vi "运维调试_五参数.vi"() -> ()   [LabVIEW 2016, in "斯坦道仪器.lvlib"]
uses:
  <vilib>/Utility/miscctls.llb/LVPointTypeDef.ctl
panel:
  out "COM口":string
  in  "打开串口":bool
  in  "释放串口":bool
  out "多参数横条运行状态":T1(xcontrol)
  in  "数据区":i32(listbox)
  in  "探头选择":u16(ring)=9 items=["氨氮"=3, "水温"=9, "pH值"=10, "溶解氧"=11, "电导率"=12, "浊度"=13, "叶绿素a"=14, "藻密度"=15, "蓝绿藻"=16, "氧化还原电位"=17, "溶解氧%"=18, "盐度"=19]
  in  "测量数据区读取":bool
  in  "测量数据区":i32(listbox)
  in  "状态告警区读取":bool
  in  "状态告警区":i32(listbox)
  in  "读取KB":bool
  in  "写入KB":bool
  out "B":dbl caption="校准值B:"
  out "K":dbl caption="校准值K:"
  in  "校准区探头选择":u16(ring)=9 items=["氨氮"=3, "水温"=9, "pH值"=10, "溶解氧"=11, "电导率"=12, "浊度"=13, "叶绿素a"=14, "藻密度"=15, "蓝绿藻"=16, "氧化还原电位"=17, "溶解氧%"=18, "盐度"=19]
  in  "停止测量(单探)":bool
  in  "启动测量(单探)":bool
  in  "控制命令区探头选择":u16(ring)=9 items=["氨氮"=3, "水温"=9, "pH值"=10, "溶解氧"=11, "电导率"=12, "浊度"=13, "叶绿素a"=14, "藻密度"=15, "蓝绿藻"=16, "氧化还原电位"=17, "溶解氧%"=18, "盐度"=19]
  in  "同步时间":bool
  in  "初始化(清洗)":bool
  in  "停止测量(全部)":bool
  in  "启动测量(全部)":bool
  in  "关键参数区读取":bool
  in  "关键参数区":i32(listbox)
  in  "传感器参数读取":bool
  in  "传感器区":i32(listbox)
  in  "返回":bool
  in  "设置":bool
  out "运行状态":string
  out "开机状态":bool
  in  "停止":bool
  in  "手动启动":bool
  out "集成报警信息":string
  # "控制命令区"
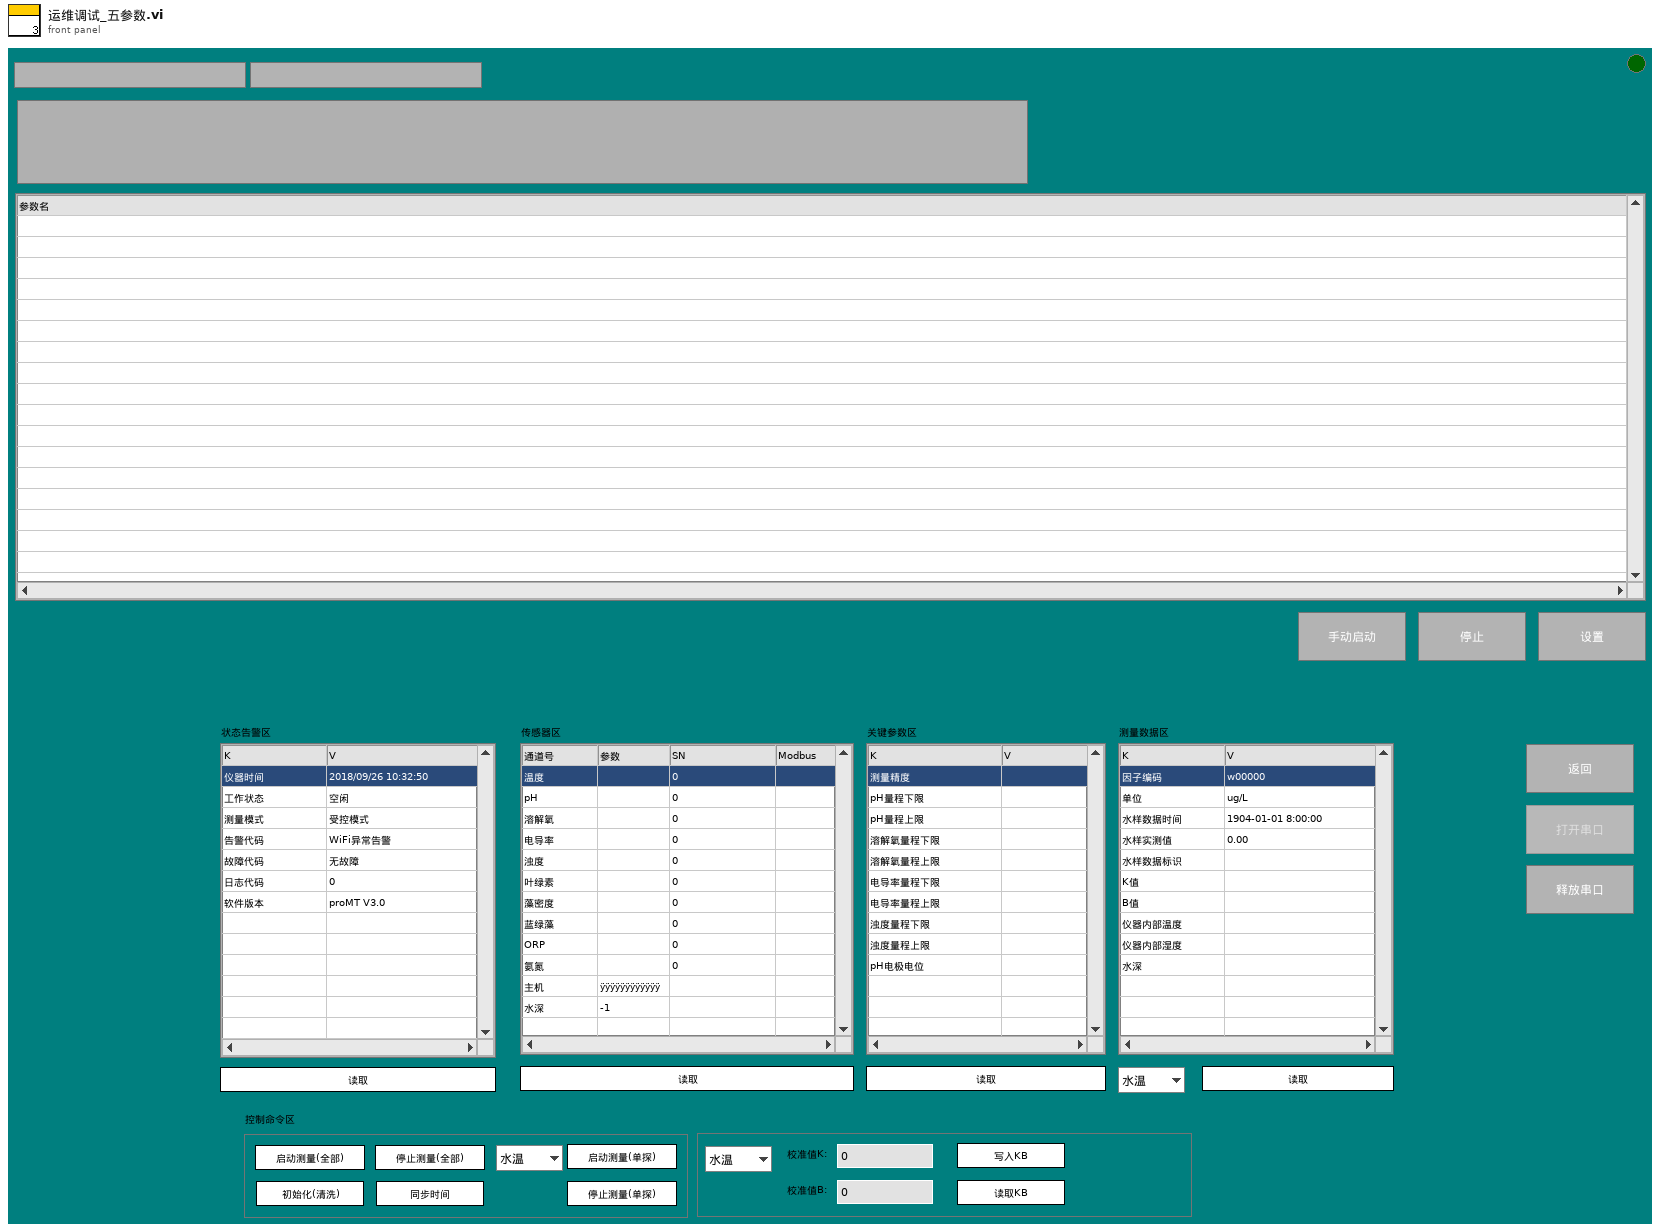
[diagram p1: front panel]
types:
  T1 = cluster{"系统时间":timestamp, "工作状态":u16, "测量模式":u16, "告警代码":enum16{"无告警", "缺试剂告警", "缺水样告警", "缺蒸馏水告警", "缺标液告警", "仪表漏液告警", "标定异常告警", "超量程告警", "加热异常", "低试剂预警", "超上限告警", "超下限告警", "仪表内部其他异常", "滴定异常告警", "电极异常告警", "量程切换告警", "参数设置告警", "PH电极电位异常", "电导率电极异常", "浊度光度异常", "溶解氧电极异常", "溶解氧光强异常", "温度异常告警", "PH异常告警", "溶解氧异常告警", "电导率异常告警", "浊度异常告警", "叶绿素异常告警", "藻密度异常告警", "蓝绿藻异常告警", "ORP异常告警", "氨氮异常告警", "清洁刷异常告警", "SD卡异常告警", "蓝牙异常告警", "Wifi异常告警", "流程异常告警"}, "故障代码":enum16{"无故障", "电机故障", "温度故障", "通讯故障", "滴定故障"}, "日志代码":u16, "软件版本":string}
  T2 = typedef "LVPointTypeDef.ctl" = cluster{"Horizontal":i16, "Vertical":i16}
  T3 = cluster{"时间标识":timestamp, "设备":string, "日志信息":string}
  T4 = enum16{"无告警", "缺试剂告警", "缺水样告警", "缺蒸馏水告警", "缺标液告警", "仪表漏液告警", "标定异常告警", "超量程告警", "加热异常", "低试剂预警", "超上限告警", "超下限告警", "仪表内部其他异常", "滴定异常告警", "电极异常告警", "量程切换告警", "参数设置告警", "PH电极电位异常", "电导率电极异常", "浊度光度异常", "溶解氧电极异常", "溶解氧光强异常", "温度异常告警", "PH异常告警", "溶解氧异常告警", "电导率异常告警", "浊度异常告警", "叶绿素异常告警", "藻密度异常告警", "蓝绿藻异常告警", "ORP异常告警", "氨氮异常告警", "清洁刷异常告警", "SD卡异常告警", "蓝牙异常告警", "Wifi异常告警", "流程异常告警"}
  T5 = cluster{"水温":dbl, "pH":dbl, "DO":dbl, "Cond":dbl, "Turb":dbl, "叶绿素":dbl, "藻密度":dbl, "蓝绿藻":dbl, "ORP":dbl, "NH3N":dbl}
  T6 = cluster{"因子编码":string, "单位":string, "标样参考值":sgl, "水样数据时间":timestamp, "水样实测值":sgl, "水样数据标识":string, "K":sgl, "B":sgl, "T":sgl, "H":sgl, "水深":sgl, "探头温度":sgl}
  T7 = enum8{"Enabled", "Disabled", "Disabled and Grayed Out"}
  T8 = cluster{"测量模式":enum16{"待机", "水样测试", "标样核查", "零点核查", "跨度核查", "空白测试", "平行样测试", "加标回收", "空白校准", "标样校准", "初始化（清洗）"}, "数据标记表":string, "测量时间":dbl}
  T9 = enum32{"Bad", "Idle", "Run top level", "Running"}
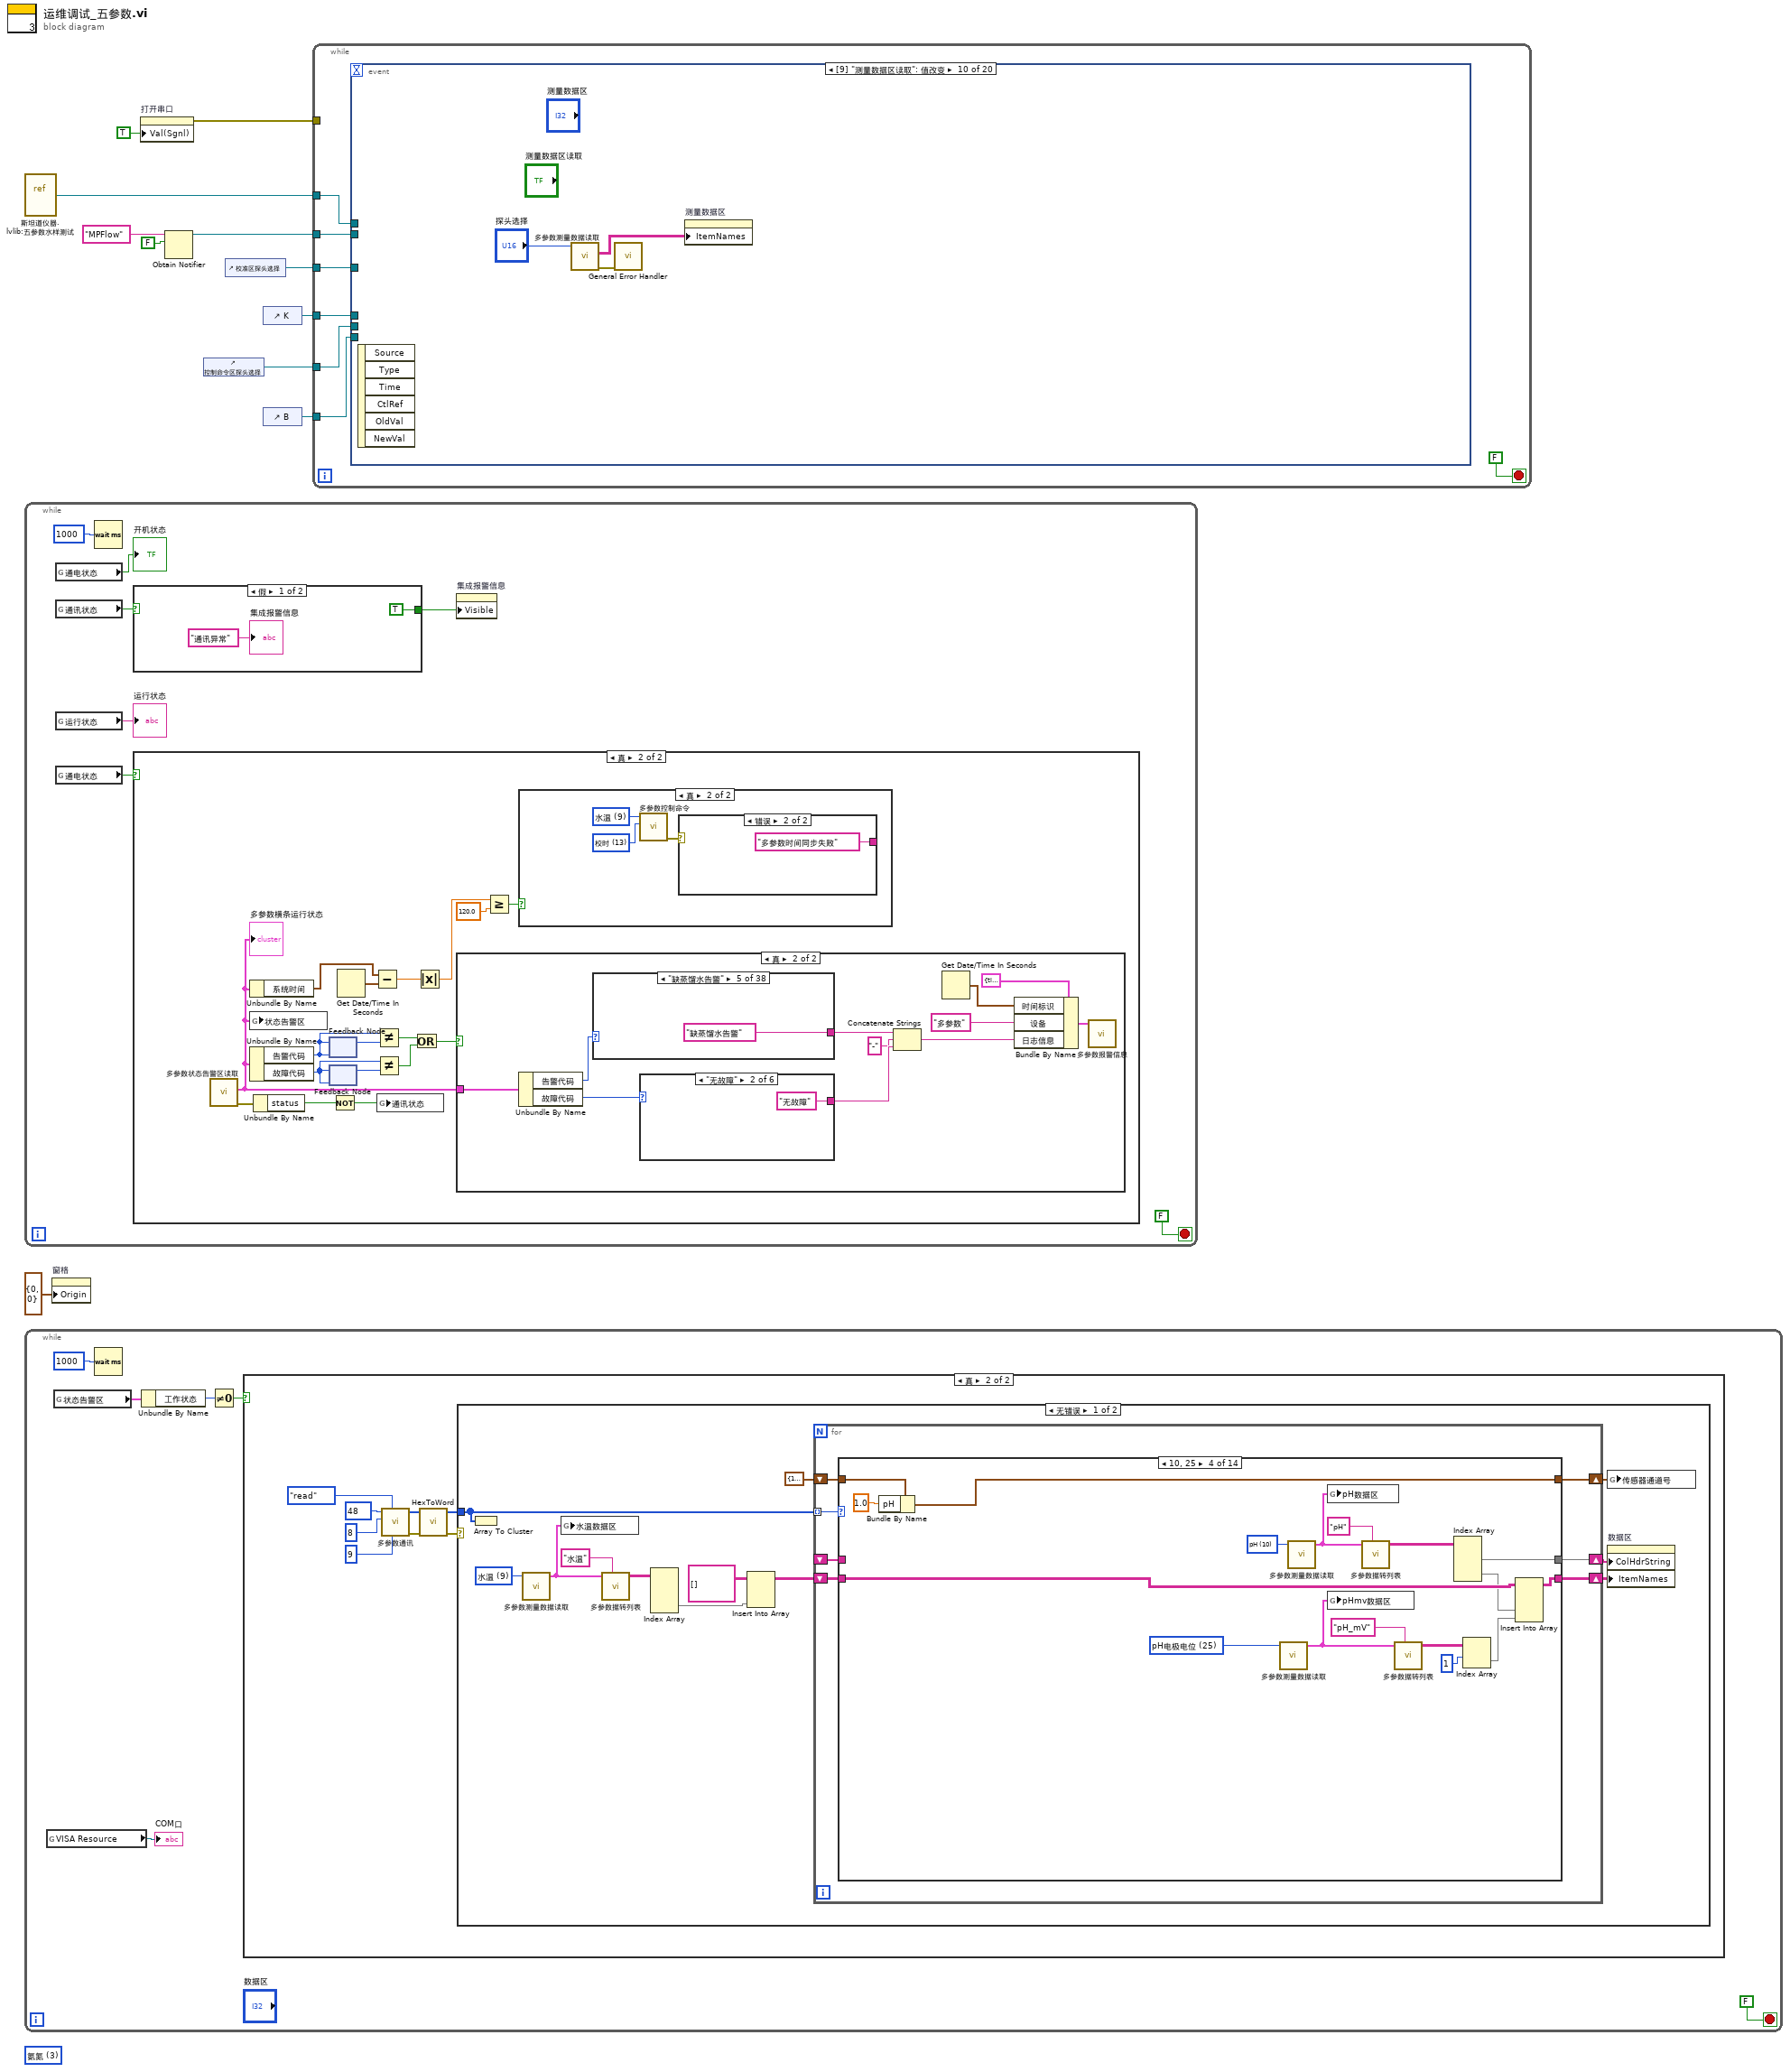
[diagram p0: block diagram]
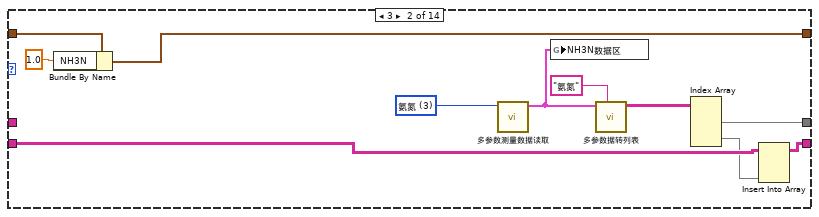
[diagram p4: hidden frame]
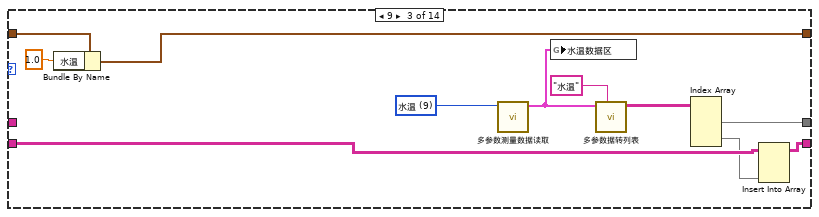
[diagram p5: hidden frame]
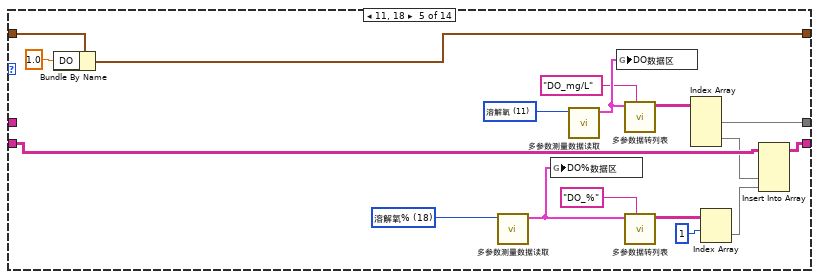
[diagram p6: hidden frame]
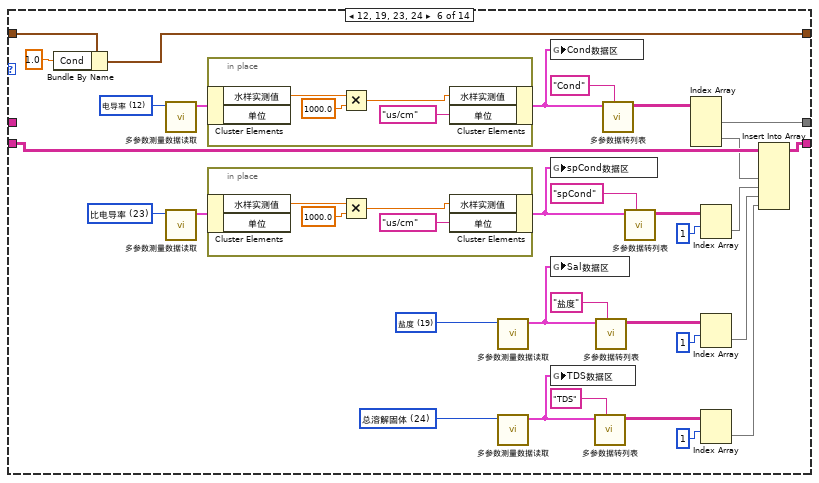
[diagram p7: hidden frame]
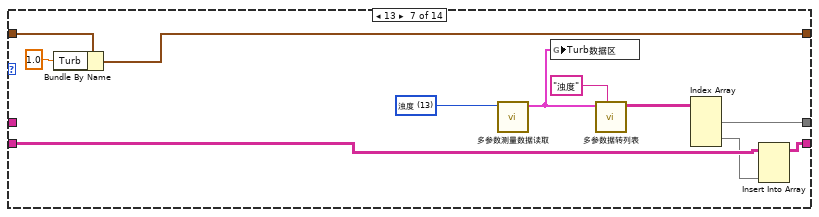
[diagram p8: hidden frame]
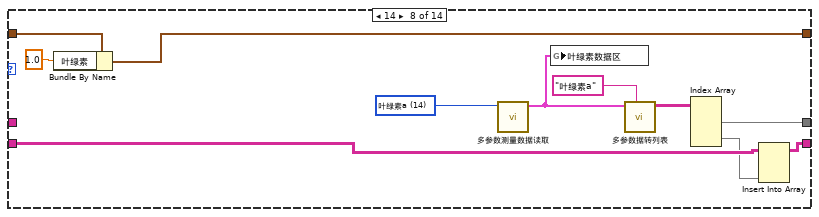
[diagram p9: hidden frame]
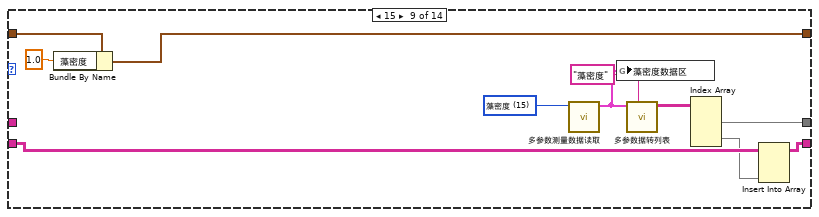
[diagram p10: hidden frame]
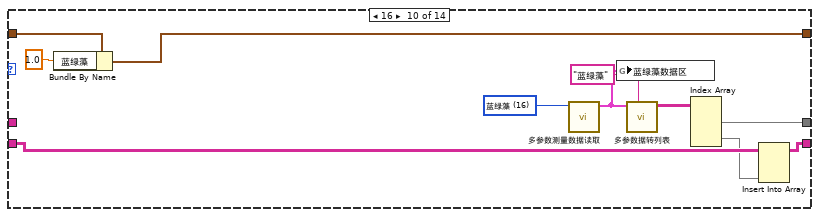
[diagram p11: hidden frame]
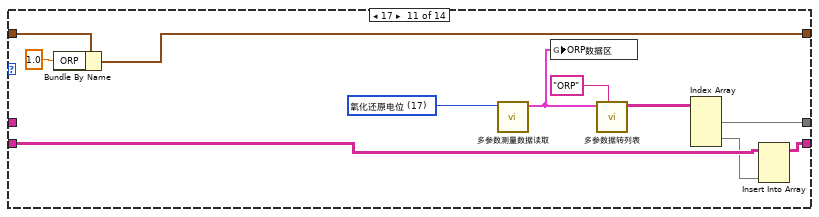
[diagram p12: hidden frame]
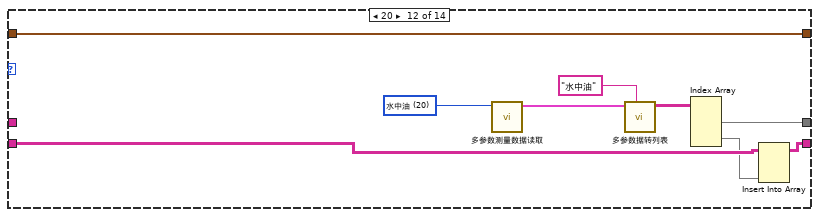
[diagram p13: hidden frame]
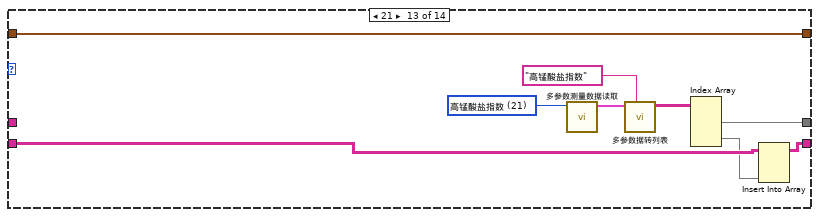
[diagram p14: hidden frame]
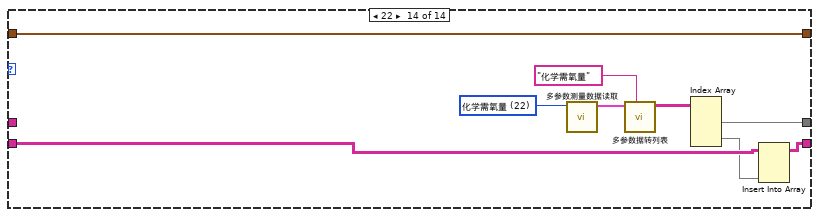
[diagram p15: hidden frame]
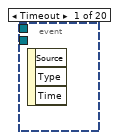
[diagram p17: hidden frame]
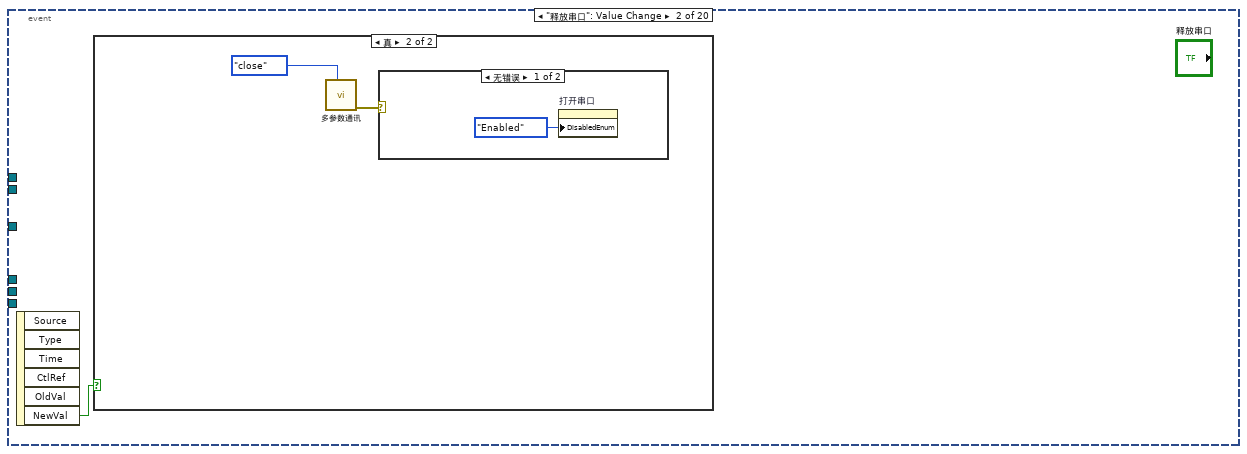
[diagram p18: hidden frame]
diagram:
  (unwired) u16 3 items=["氨氮"=3, "水温"=9, "pH"=10, "溶解氧"=11, "电导率"=12, "浊度"=13, "叶绿素a"=14, "藻密度"=15, "蓝绿藻"=16, "氧化还原电位"=17, "溶解氧%"=18, "盐度"=19, "水中油"=20, "高锰酸盐指数"=21, "化学需氧量"=22, "比电导率"=23, "总溶解固体"=24, "pH电极电位"=25] ("下拉列表")
  n1 = vi-ref "斯坦道仪器.lvlib:五参数水样测试.vi"() -> (w8:refnum<vi>)
  n2 = while {
    stop <- FALSE stop-if-true
    n3 = global read "多参数全局变量.vi" "通电状态"() -> (→"开机状态":bool)
    n4 = global read "多参数全局变量.vi" "通讯状态"() -> (w16:bool)
    n5 = global read "多参数全局变量.vi" "运行状态"() -> (→"运行状态":string)
    n6 = global read "多参数全局变量.vi" "通电状态"() -> (w12:bool)
    n7 = Wait (ms)(milliseconds to wait=u32 1000 ("等待时间（毫秒）")) -> ()  [unwired: 1 out]
    n8 = case shown="假" w16 {
      tunnel: [TRUE ("可见") _] -> w15
      frame False {
        "集成报警信息" <- "通讯异常" ("集成报警信息")
      }
      frame True {
      }
    }
    n9 = case shown="真" w12 {
      frame False {
      }
      frame True {
        n10 = call "多参数状态告警区读取.vi"() -> ("error out"=w28:errorcluster, "状态告警块"=w25:T1)  [unwired: 9 in, 1 out]
        "多参数横条运行状态" <- w25
        n11 = Unbundle By Name(w25) -> ("系统时间"=w24:timestamp)
        n12 = global write "多参数全局变量.vi" "状态告警区"(w25) -> ()
        n13 = Unbundle By Name(w25) -> ("告警代码"=w34:T4, "故障代码"=w32:enum16{"无故障", "电机故障", "温度故障", "通讯故障", "滴定故障"})
        n14 = Unbundle By Name(w28) -> ("status"=w27:bool)
        n15 = feedback #1(w34) -> (w35:T4)
        n16 = feedback-in #1(w34) -> ()
        n17 = feedback #2(w32) -> (w33:enum16{"无故障", "电机故障", "温度故障", "通讯故障", "滴定故障"})
        n18 = feedback-in #2(w32) -> ()
        n19 = Not(x=w27) -> (.not. x?=w26:bool)
        n20 = Get Date/Time In Seconds() -> (seconds since 1Jan1904=w23:timestamp)
        n21 = Subtract(x=w24, y=w23) -> (x-y=w22:dbl)
        n22 = Not Equal?(x=w34, y=w35) -> (x != y?=w30:bool)
        n23 = Not Equal?(x=w32, y=w33) -> (x != y?=w31:bool)
        n24 = global write "多参数全局变量.vi" "通讯状态"(w26) -> ()
        n25 = Or(x=w30, y=w31) -> (x .or. y?=w29:bool)
        n26 = Absolute Value(x=w22) -> (abs(x)=w21:dbl)
        n27 = case shown="真" w29 {
          tunnel: w25 -> [_ w51]
          frame False {
          }
          frame True {
            n28 = Unbundle By Name(w51) -> ("告警代码"=w50:T4, "故障代码"=w49:enum16{"无故障", "电机故障", "温度故障", "通讯故障", "滴定故障"})
            n29 = case shown="\"缺蒸馏水告警\"" w50 {
              selector: w50 -> [w62 _ _ _ _ _ _ _ _ _ _ _ _ _ _ _ _ _ _ _ _ _ _ _ _ _ _ _ _ _ _ _ _ _ _ _ _ _]
              tunnel: [w61 "无告警" "缺试剂告警" "缺水样告警" "缺蒸馏水告警" "缺标液告警" "仪表漏液告警" "标定异常告警" "超量程告警" "加热异常" "低试剂预警" "超上限告警" "超下限告警" "仪表内部其他异常" "滴定异常告警" "电极异常告警" "量程切换告警" "参数设置告警" "PH电极电位异常" "电导率电极异常" "浊度光度异常" "溶解氧电极异常" "溶解氧光强异常" "温度异常告警" "PH异常告警" "溶解氧异常告警" "电导率异常告警" "浊度异常告警" "叶绿素异常告警" "藻密度异常告警" "蓝绿藻异常告警" "ORP异常告警" "氨氮异常告警" "清洁刷异常告警" "SD卡异常告警" "蓝牙异常告警" "WiFi异常告警" "流程异常告警"] -> w48
              frame Default {
                n30 = Format Into String(format string="%d" ("格式字符串"), initial string="未知" ("工作状态"), w62) -> (resulting string=w61:string)  [unwired: 1 in, 1 out]
              }
              frame "无告警" {
              }
              frame "缺试剂告警" {
              }
              frame "缺水样告警" {
              }
              frame "缺蒸馏水告警" {
              }
              frame "缺标液告警" {
              }
              frame "仪表漏液告警" {
              }
              frame "标定异常告警" {
              }
              frame "超量程告警" {
              }
              frame "加热异常" {
              }
              frame "低试剂预警" {
              }
              frame "超上限告警" {
              }
              frame "超下限告警" {
              }
              frame "仪表内部其他异常" {
              }
              frame "滴定异常告警" {
              }
              frame "电极异常告警" {
              }
              frame "量程切换告警" {
              }
              frame "参数设置告警" {
              }
              frame "PH电极电位异常" {
              }
              frame "电导率电极异常" {
              }
              frame "浊度光度异常" {
              }
              frame "溶解氧电极异常" {
              }
              frame "溶解氧光强异常" {
              }
              frame "温度异常告警" {
              }
              frame "PH异常告警" {
              }
              frame "溶解氧异常告警" {
              }
              frame "电导率异常告警" {
              }
              frame "浊度异常告警" {
              }
              frame "叶绿素异常告警" {
              }
              frame "藻密度异常告警" {
              }
              frame "蓝绿藻异常告警" {
              }
              frame "ORP异常告警" {
              }
              frame "氨氮异常告警" {
              }
              frame "清洁刷异常告警" {
              }
              frame "SD卡异常告警" {
              }
              frame "蓝牙异常告警" {
              }
              frame "Wifi异常告警" {
              }
              frame "流程异常告警" {
              }
            }
            n31 = case shown="\"无故障\"" w49 {
              selector: w49 -> [w53 _ _ _ _ _]
              tunnel: [w52 "无故障" "电机故障" "温度故障" "通讯故障" "滴定故障"] -> w47
              frame Default {
                n32 = Format Into String(format string="%d" ("格式字符串"), initial string="未知" ("工作状态"), w53) -> (resulting string=w52:string)  [unwired: 1 in, 1 out]
              }
              frame "无故障" {
              }
              frame "电机故障" {
              }
              frame "温度故障" {
              }
              frame "通讯故障" {
              }
              frame "滴定故障" {
              }
            }
            n33 = Concatenate Strings(w48, "-" ("字符串"), w47) -> (w43:string)
            n34 = Get Date/Time In Seconds() -> (seconds since 1Jan1904=w42:timestamp)
            n35 = Bundle By Name(cluster=T3 {"时间标识"=timestamp(0 s since 1904-01-01), "设备"="", "日志信息"=""} ("data in"), "时间标识"=w42, "设备"="多参数", "日志信息"=w43) -> (w44:T3)
            n36 = call "多参数报警信息.vi"("data in"=w44) -> ()  [unwired: 10 in, 1 out]
          }
        }
        n37 = Greater Or Equal?(x=w21, y=120.0) -> (x >= y?=w20:bool)
        n38 = case shown="真" w20 {
          frame False {
          }
          frame True {
            w36 = u16 13 items=["启动测量（全部）"=1, "初始化（清洗）"=10, "停止测量（全部）"=11, "校时"=13, "启动测量（单个传感器）"=19, "停止测量（单个传感器）"=20] ("控制命令")
            w37 = u16 9 items=["氨氮"=3, "水温"=9, "pH值"=10, "溶解氧"=11, "电导率"=12, "浊度"=13, "叶绿素a"=14, "藻密度"=15, "蓝绿藻"=16, "氧化还原电位"=17, "溶解氧%"=18, "盐度"=19] ("站号")
            n39 = call "多参数控制命令.vi"("控制命令"=w36, "站号"=w37) -> ("error out"=w38:errorcluster)  [unwired: 9 in]
            n40 = case shown="错误" w38 {
              tunnel: ["多参数时间同步成功" ("消息") "多参数时间同步失败" ("消息")] -> _
              frame No Error {
              }
              frame Error {
              }
            }
          }
        }
      }
    }
    n41 = property on="集成报警信息" class="Str"("Visible"=w15) -> ()  [unwired: 2 in, 2 out]
  }
  n42 = while {
    stop <- FALSE stop-if-true
    n43 = global read "多参数全局变量.vi" "VISA Resource"() -> (→"COM口":refnum<visa-resource-name>)
    n44 = global read "多参数全局变量.vi" "状态告警区"() -> (w107:T1)
    n45 = Wait (ms)(milliseconds to wait=u32 1000 ("等待时间（毫秒）")) -> ()  [unwired: 1 out]
    n46 = Unbundle By Name(w107) -> ("工作状态"=w106:u16)
    n47 = Not Equal To 0?(x=w106) -> (x != 0?=w105:bool)
    n48 = case shown="真" w105 {
      frame False {
      }
      frame True {
        n49 = call "多参数通讯.vi"("Slave ID"=u8 9, "STEP"=enum16{"open", "read", "write", "close"}."read", "quantity"=u16 8, "starting address"=u16 48) -> ("error out"=w112:errorcluster, "Registers"=w113:u16[])  [unwired: 5 in, 1 out]
        n50 = call "HexToWord.vi"("数组"=w113) -> ("WORD"=w116:u16[])  [unwired: 10 in]
        n51 = case shown="无错误" w112 {
          tunnel: w116 -> [w128 _]
          frame No Error {
            w125 = u16 9 items=["氨氮"=3, "水温"=9, "pH"=10, "溶解氧"=11, "电导率"=12, "浊度"=13, "叶绿素a"=14, "藻密度"=15, "蓝绿藻"=16, "氧化还原电位"=17, "溶解氧%"=18, "盐度"=19, "水中油"=20, "高锰酸盐指数"=21, "化学需氧量"=22, "比电导率"=23, "总溶解固体"=24, "pH电极电位"=25] ("下拉列表")
            n52 = Array To Cluster(array=w128) -> ()  [unwired: 1 out]
            n53 = call "多参数测量数据读取.vi"("探头选择"=w125) -> ("测量数据块"=w120:T6)  [unwired: 8 in, 2 out]
            n54 = global write "多参数全局变量.vi" "水温数据区"(w120) -> ()
            n55 = call "多参数据转列表.vi"("参数名"="水温", "测量数据块"=w120) -> ("添加的数组"=w118:string[][])  [unwired: 9 in]
            n56 = Index Array(array=w118) -> (element #2=w117:string[])  [unwired: 4 in, 1 out]
            n57 = Insert Into Array(array=string[][] [] ("子数组"), new element=w117) -> (w123:string[][])  [unwired: 2 in]
            n58 = for {
              tunnel: w128 -> [w135] mode=indexing
              shift-right: [w133] -> w126
              shift-left: w123 -> [w134]
              shift-right: [w132] -> w127
              shift-left: _ -> [w131]
              shift-right: [w130] -> w121
              shift-left: T5 {"水温"=1.0, "pH"=0.0, "DO"=0.0, "Cond"=0.0, "Turb"=0.0, "叶绿素"=0.0, "藻密度"=0.0, "蓝绿藻"=0.0, "ORP"=0.0, "NH3N"=0.0} ("传感器通道号") -> [w129]
              n59 = case shown="10, 25" w135 {
                tunnel: w134 -> [w138 w148 w159 w176 w193 w224 w243 w254 w265 w276 w287 w296 w305 w314]
                tunnel: [w138 w147 w158 w175 w192 w223 w242 w253 w264 w275 w286 w295 w304 w313] -> w133
                tunnel: [w137 w140 w151 w168 w185 w214 w236 w246 w259 w269 w280 w290 w299 w308] -> w132
                tunnel: w131 -> [w137 _ _ _ _ _ _ _ _ _ _ _ _ _]
                tunnel: [w136 w144 w155 w171 w189 w217 w239 w250 w261 w272 w283 w294 w303 w312] -> w130
                tunnel: w129 -> [w136 w146 w157 w173 w191 w218 w240 w251 w262 w273 w284 w294 w303 w312]
                frame 0, Default {
                }
                frame 3 {
                  w149 = u16 3 items=["氨氮"=3, "水温"=9, "pH"=10, "溶解氧"=11, "电导率"=12, "浊度"=13, "叶绿素a"=14, "藻密度"=15, "蓝绿藻"=16, "氧化还原电位"=17, "溶解氧%"=18, "盐度"=19, "水中油"=20, "高锰酸盐指数"=21, "化学需氧量"=22, "比电导率"=23, "总溶解固体"=24, "pH电极电位"=25] ("下拉列表")
                  n60 = Bundle By Name(cluster=w146, "NH3N"=1.0) -> (w144:T5)
                  n61 = call "多参数测量数据读取.vi"("探头选择"=w149) -> ("测量数据块"=w143:T6)  [unwired: 8 in, 2 out]
                  n62 = global write "多参数全局变量.vi" "NH3N数据区"(w143) -> ()
                  n63 = call "多参数据转列表.vi"("参数名"="氨氮", "测量数据块"=w143) -> ("添加的数组"=w142:string[][])  [unwired: 9 in]
                  n64 = Index Array(array=w142) -> (element #1=w140:string[], element #2=w139:string[])  [unwired: 4 in]
                  n65 = Insert Into Array(array=w148, new element=w139) -> (w147:string[][])  [unwired: 2 in]
                }
                frame 9 {
                  w160 = u16 9 items=["氨氮"=3, "水温"=9, "pH"=10, "溶解氧"=11, "电导率"=12, "浊度"=13, "叶绿素a"=14, "藻密度"=15, "蓝绿藻"=16, "氧化还原电位"=17, "溶解氧%"=18, "盐度"=19, "水中油"=20, "高锰酸盐指数"=21, "化学需氧量"=22, "比电导率"=23, "总溶解固体"=24, "pH电极电位"=25] ("下拉列表")
                  n66 = Bundle By Name(cluster=w157, "水温"=1.0) -> (w155:T5)
                  n67 = call "多参数测量数据读取.vi"("探头选择"=w160) -> ("测量数据块"=w154:T6)  [unwired: 8 in, 2 out]
                  n68 = global write "多参数全局变量.vi" "水温数据区"(w154) -> ()
                  n69 = call "多参数据转列表.vi"("参数名"="水温", "测量数据块"=w154) -> ("添加的数组"=w153:string[][])  [unwired: 9 in]
                  n70 = Index Array(array=w153) -> (element #1=w151:string[], element #2=w150:string[])  [unwired: 4 in]
                  n71 = Insert Into Array(array=w159, new element=w150) -> (w158:string[][])  [unwired: 2 in]
                }
                frame 10, 25 {
                  w174 = u16 25 items=["氨氮"=3, "水温"=9, "pH"=10, "溶解氧"=11, "电导率"=12, "浊度"=13, "叶绿素a"=14, "藻密度"=15, "蓝绿藻"=16, "氧化还原电位"=17, "溶解氧%"=18, "盐度"=19, "水中油"=20, "高锰酸盐指数"=21, "化学需氧量"=22, "比电导率"=23, "总溶解固体"=24, "pH电极电位"=25] ("下拉列表")
                  w177 = u16 10 items=["氨氮"=3, "水温"=9, "pH"=10, "溶解氧"=11, "电导率"=12, "浊度"=13, "叶绿素a"=14, "藻密度"=15, "蓝绿藻"=16, "氧化还原电位"=17, "溶解氧%"=18, "盐度"=19, "水中油"=20, "高锰酸盐指数"=21, "化学需氧量"=22, "比电导率"=23, "总溶解固体"=24, "pH电极电位"=25] ("下拉列表")
                  n72 = Bundle By Name(cluster=w173, "pH"=1.0) -> (w171:T5)
                  n73 = call "多参数测量数据读取.vi"("探头选择"=w174) -> ("测量数据块"=w164:T6)  [unwired: 8 in, 2 out]
                  n74 = call "多参数测量数据读取.vi"("探头选择"=w177) -> ("测量数据块"=w170:T6)  [unwired: 8 in, 2 out]
                  n75 = global write "多参数全局变量.vi" "pH数据区"(w170) -> ()
                  n76 = global write "多参数全局变量.vi" "pHmv数据区"(w164) -> ()
                  n77 = call "多参数据转列表.vi"("参数名"="pH", "测量数据块"=w170) -> ("添加的数组"=w169:string[][])  [unwired: 9 in]
                  n78 = call "多参数据转列表.vi"("参数名"="pH_mV", "测量数据块"=w164) -> ("添加的数组"=w163:string[][])  [unwired: 9 in]
                  n79 = Index Array(array=w169) -> (element #1=w168:string[], element #2=w167:string[])  [unwired: 4 in]
                  n80 = Index Array(array=w163, index (row)=1 ("禁用的索引 (列)")) -> (element=w166:string[])  [unwired: 1 in]
                  n81 = Insert Into Array(array=w176, new element #1=w167, new element #2=w166) -> (w175:string[][])  [unwired: 2 in]
                }
                frame 11, 18 {
                  w183 = u16 18 items=["氨氮"=3, "水温"=9, "pH"=10, "溶解氧"=11, "电导率"=12, "浊度"=13, "叶绿素a"=14, "藻密度"=15, "蓝绿藻"=16, "氧化还原电位"=17, "溶解氧%"=18, "盐度"=19, "水中油"=20, "高锰酸盐指数"=21, "化学需氧量"=22, "比电导率"=23, "总溶解固体"=24, "pH电极电位"=25] ("下拉列表")
                  w194 = u16 11 items=["氨氮"=3, "水温"=9, "pH"=10, "溶解氧"=11, "电导率"=12, "浊度"=13, "叶绿素a"=14, "藻密度"=15, "蓝绿藻"=16, "氧化还原电位"=17, "溶解氧%"=18, "盐度"=19, "水中油"=20, "高锰酸盐指数"=21, "化学需氧量"=22, "比电导率"=23, "总溶解固体"=24, "pH电极电位"=25] ("下拉列表")
                  n82 = Bundle By Name(cluster=w191, "DO"=1.0) -> (w189:T5)
                  n83 = call "多参数测量数据读取.vi"("探头选择"=w183) -> ("测量数据块"=w182:T6)  [unwired: 8 in, 2 out]
                  n84 = global write "多参数全局变量.vi" "DO%数据区"(w182) -> ()
                  n85 = call "多参数测量数据读取.vi"("探头选择"=w194) -> ("测量数据块"=w188:T6)  [unwired: 8 in, 2 out]
                  n86 = global write "多参数全局变量.vi" "DO数据区"(w188) -> ()
                  n87 = call "多参数据转列表.vi"("参数名"="DO_mg/L", "测量数据块"=w188) -> ("添加的数组"=w186:string[][])  [unwired: 9 in]
                  n88 = call "多参数据转列表.vi"("参数名"="DO_%", "测量数据块"=w182) -> ("添加的数组"=w180:string[][])  [unwired: 9 in]
                  n89 = Index Array(array=w186) -> (element #1=w185:string[], element #2=w184:string[])  [unwired: 4 in]
                  n90 = Index Array(array=w180, index (row)=1 ("禁用的索引 (列)")) -> (element=w179:string[])  [unwired: 1 in]
                  n91 = Insert Into Array(array=w193, new element #1=w184, new element #2=w179) -> (w192:string[][])  [unwired: 2 in]
                }
                frame 12, 19, 23, 24 {
                  w220 = u16 24 items=["氨氮"=3, "水温"=9, "pH"=10, "溶解氧"=11, "电导率"=12, "浊度"=13, "叶绿素a"=14, "藻密度"=15, "蓝绿藻"=16, "氧化还原电位"=17, "溶解氧%"=18, "盐度"=19, "水中油"=20, "高锰酸盐指数"=21, "化学需氧量"=22, "比电导率"=23, "总溶解固体"=24, "pH电极电位"=25] ("下拉列表")
                  w221 = u16 19 items=["氨氮"=3, "水温"=9, "pH"=10, "溶解氧"=11, "电导率"=12, "浊度"=13, "叶绿素a"=14, "藻密度"=15, "蓝绿藻"=16, "氧化还原电位"=17, "溶解氧%"=18, "盐度"=19, "水中油"=20, "高锰酸盐指数"=21, "化学需氧量"=22, "比电导率"=23, "总溶解固体"=24, "pH电极电位"=25] ("下拉列表")
                  w222 = u16 23 items=["氨氮"=3, "水温"=9, "pH"=10, "溶解氧"=11, "电导率"=12, "浊度"=13, "叶绿素a"=14, "藻密度"=15, "蓝绿藻"=16, "氧化还原电位"=17, "溶解氧%"=18, "盐度"=19, "水中油"=20, "高锰酸盐指数"=21, "化学需氧量"=22, "比电导率"=23, "总溶解固体"=24, "pH电极电位"=25] ("下拉列表")
                  w225 = u16 12 items=["氨氮"=3, "水温"=9, "pH"=10, "溶解氧"=11, "电导率"=12, "浊度"=13, "叶绿素a"=14, "藻密度"=15, "蓝绿藻"=16, "氧化还原电位"=17, "溶解氧%"=18, "盐度"=19, "水中油"=20, "高锰酸盐指数"=21, "化学需氧量"=22, "比电导率"=23, "总溶解固体"=24, "pH电极电位"=25] ("下拉列表")
                  n92 = Bundle By Name(cluster=w218, "Cond"=1.0 ("DO")) -> (w217:T5)
                  n93 = call "多参数测量数据读取.vi"("探头选择"=w225) -> ("测量数据块"=w201:T6)  [unwired: 8 in, 2 out]
                  n94 = call "多参数测量数据读取.vi"("探头选择"=w222) -> ("测量数据块"=w199:T6)  [unwired: 8 in, 2 out]
                  n95 = in-place {
                    n96 = in-place-cluster #3(w201) -> ("水样实测值"=w232:sgl)  [unwired: 1 out]
                    n97 = Multiply(x=w232, y=sgl 1000.0) -> (x*y=w230:sgl)
                    n98 = in-place-cluster #3("水样实测值"=w230, "单位"="us/cm") -> (w200:T6)
                  }
                  n99 = in-place {
                    n100 = in-place-cluster #4(w199) -> ("水样实测值"=w228:sgl)  [unwired: 1 out]
                    n101 = Multiply(x=w228, y=sgl 1000.0) -> (x*y=w226:sgl)
                    n102 = in-place-cluster #4("水样实测值"=w226, "单位"="us/cm") -> (w198:T6)
                  }
                  n103 = call "多参数测量数据读取.vi"("探头选择"=w221) -> ("测量数据块"=w208:T6)  [unwired: 8 in, 2 out]
                  n104 = call "多参数测量数据读取.vi"("探头选择"=w220) -> ("测量数据块"=w204:T6)  [unwired: 8 in, 2 out]
                  n105 = global write "多参数全局变量.vi" "Cond数据区"(w200) -> ()
                  n106 = global write "多参数全局变量.vi" "spCond数据区"(w198) -> ()
                  n107 = global write "多参数全局变量.vi" "Sal数据区"(w208) -> ()
                  n108 = global write "多参数全局变量.vi" "TDS数据区"(w204) -> ()
                  n109 = call "多参数据转列表.vi"("参数名"="TDS", "测量数据块"=w204) -> ("添加的数组"=w203:string[][])  [unwired: 9 in]
                  n110 = call "多参数据转列表.vi"("参数名"="盐度", "测量数据块"=w208) -> ("添加的数组"=w207:string[][])  [unwired: 9 in]
                  n111 = call "多参数据转列表.vi"("参数名"="Cond", "测量数据块"=w200) -> ("添加的数组"=w215:string[][])  [unwired: 9 in]
                  n112 = call "多参数据转列表.vi"("参数名"="spCond", "测量数据块"=w198) -> ("添加的数组"=w211:string[][])  [unwired: 9 in]
                  n113 = Index Array(array=w215) -> (element #1=w214:string[], element #2=w213:string[])  [unwired: 4 in]
                  n114 = Index Array(array=w211, index (row)=1 ("禁用的索引 (列)")) -> (element=w210:string[])  [unwired: 1 in]
                  n115 = Index Array(array=w207, index (row)=1 ("禁用的索引 (列)")) -> (element=w206:string[])  [unwired: 1 in]
                  n116 = Index Array(array=w203, index (row)=1 ("禁用的索引 (列)")) -> (element=w202:string[])  [unwired: 1 in]
                  n117 = Insert Into Array(array=w224, new element #1=w213, new element #2=w210, new element #3=w206, new element #4=w202) -> (w223:string[][])  [unwired: 2 in]
                }
                frame 13 {
                  w244 = u16 13 items=["氨氮"=3, "水温"=9, "pH"=10, "溶解氧"=11, "电导率"=12, "浊度"=13, "叶绿素a"=14, "藻密度"=15, "蓝绿藻"=16, "氧化还原电位"=17, "溶解氧%"=18, "盐度"=19, "水中油"=20, "高锰酸盐指数"=21, "化学需氧量"=22, "比电导率"=23, "总溶解固体"=24, "pH电极电位"=25] ("下拉列表")
                  n118 = Bundle By Name(cluster=w240, "Turb"=1.0 ("DO")) -> (w239:T5)
                  n119 = call "多参数测量数据读取.vi"("探头选择"=w244) -> ("测量数据块"=w234:T6)  [unwired: 8 in, 2 out]
                  n120 = global write "多参数全局变量.vi" "Turb数据区"(w234) -> ()
                  n121 = call "多参数据转列表.vi"("参数名"="浊度", "测量数据块"=w234) -> ("添加的数组"=w237:string[][])  [unwired: 9 in]
                  n122 = Index Array(array=w237) -> (element #1=w236:string[], element #2=w235:string[])  [unwired: 4 in]
                  n123 = Insert Into Array(array=w243, new element=w235) -> (w242:string[][])  [unwired: 2 in]
                }
                frame 14 {
                  w255 = u16 14 items=["氨氮"=3, "水温"=9, "pH"=10, "溶解氧"=11, "电导率"=12, "浊度"=13, "叶绿素a"=14, "藻密度"=15, "蓝绿藻"=16, "氧化还原电位"=17, "溶解氧%"=18, "盐度"=19, "水中油"=20, "高锰酸盐指数"=21, "化学需氧量"=22, "比电导率"=23, "总溶解固体"=24, "pH电极电位"=25] ("下拉列表")
                  n124 = Bundle By Name(cluster=w251, "叶绿素"=1.0 ("DO")) -> (w250:T5)
                  n125 = call "多参数测量数据读取.vi"("探头选择"=w255) -> ("测量数据块"=w249:T6)  [unwired: 8 in, 2 out]
                  n126 = global write "多参数全局变量.vi" "叶绿素数据区"(w249) -> ()
                  n127 = call "多参数据转列表.vi"("参数名"="叶绿素a", "测量数据块"=w249) -> ("添加的数组"=w247:string[][])  [unwired: 9 in]
                  n128 = Index Array(array=w247) -> (element #1=w246:string[], element #2=w245:string[])  [unwired: 4 in]
                  n129 = Insert Into Array(array=w254, new element=w245) -> (w253:string[][])  [unwired: 2 in]
                }
                frame 15 {
                  w266 = u16 15 items=["氨氮"=3, "水温"=9, "pH"=10, "溶解氧"=11, "电导率"=12, "浊度"=13, "叶绿素a"=14, "藻密度"=15, "蓝绿藻"=16, "氧化还原电位"=17, "溶解氧%"=18, "盐度"=19, "水中油"=20, "高锰酸盐指数"=21, "化学需氧量"=22, "比电导率"=23, "总溶解固体"=24, "pH电极电位"=25] ("下拉列表")
                  n130 = Bundle By Name(cluster=w262, "藻密度"=1.0 ("DO")) -> (w261:T5)
                  n131 = call "多参数测量数据读取.vi"("探头选择"=w266) -> ("测量数据块"=w258:T6)  [unwired: 8 in, 2 out]
                  n132 = global write "多参数全局变量.vi" "藻密度数据区"(w258) -> ()
                  n133 = call "多参数据转列表.vi"("参数名"="藻密度", "测量数据块"=w258) -> ("添加的数组"=w260:string[][])  [unwired: 9 in]
                  n134 = Index Array(array=w260) -> (element #1=w259:string[], element #2=w257:string[])  [unwired: 4 in]
                  n135 = Insert Into Array(array=w265, new element=w257) -> (w264:string[][])  [unwired: 2 in]
                }
                frame 16 {
                  w277 = u16 16 items=["氨氮"=3, "水温"=9, "pH"=10, "溶解氧"=11, "电导率"=12, "浊度"=13, "叶绿素a"=14, "藻密度"=15, "蓝绿藻"=16, "氧化还原电位"=17, "溶解氧%"=18, "盐度"=19, "水中油"=20, "高锰酸盐指数"=21, "化学需氧量"=22, "比电导率"=23, "总溶解固体"=24, "pH电极电位"=25] ("下拉列表")
                  n136 = Bundle By Name(cluster=w273, "蓝绿藻"=1.0 ("DO")) -> (w272:T5)
                  n137 = call "多参数测量数据读取.vi"("探头选择"=w277) -> ("测量数据块"=w271:T6)  [unwired: 8 in, 2 out]
                  n138 = global write "多参数全局变量.vi" "蓝绿藻数据区"(w271) -> ()
                  n139 = call "多参数据转列表.vi"("参数名"="蓝绿藻", "测量数据块"=w271) -> ("添加的数组"=w270:string[][])  [unwired: 9 in]
                  n140 = Index Array(array=w270) -> (element #1=w269:string[], element #2=w268:string[])  [unwired: 4 in]
                  n141 = Insert Into Array(array=w276, new element=w268) -> (w275:string[][])  [unwired: 2 in]
                }
                frame 17 {
                  w288 = u16 17 items=["氨氮"=3, "水温"=9, "pH"=10, "溶解氧"=11, "电导率"=12, "浊度"=13, "叶绿素a"=14, "藻密度"=15, "蓝绿藻"=16, "氧化还原电位"=17, "溶解氧%"=18, "盐度"=19, "水中油"=20, "高锰酸盐指数"=21, "化学需氧量"=22, "比电导率"=23, "总溶解固体"=24, "pH电极电位"=25] ("下拉列表")
                  n142 = Bundle By Name(cluster=w284, "ORP"=1.0 ("DO")) -> (w283:T5)
                  n143 = call "多参数测量数据读取.vi"("探头选择"=w288) -> ("测量数据块"=w282:T6)  [unwired: 8 in, 2 out]
                  n144 = global write "多参数全局变量.vi" "ORP数据区"(w282) -> ()
                  n145 = call "多参数据转列表.vi"("参数名"="ORP", "测量数据块"=w282) -> ("添加的数组"=w281:string[][])  [unwired: 9 in]
                  n146 = Index Array(array=w281) -> (element #1=w280:string[], element #2=w278:string[])  [unwired: 4 in]
                  n147 = Insert Into Array(array=w287, new element=w278) -> (w286:string[][])  [unwired: 2 in]
                }
                frame 20 {
                  w297 = u16 20 items=["氨氮"=3, "水温"=9, "pH"=10, "溶解氧"=11, "电导率"=12, "浊度"=13, "叶绿素a"=14, "藻密度"=15, "蓝绿藻"=16, "氧化还原电位"=17, "溶解氧%"=18, "盐度"=19, "水中油"=20, "高锰酸盐指数"=21, "化学需氧量"=22, "比电导率"=23, "总溶解固体"=24, "pH电极电位"=25] ("下拉列表")
                  n148 = call "多参数测量数据读取.vi"("探头选择"=w297) -> ("测量数据块"=w293:T6)  [unwired: 8 in, 2 out]
                  n149 = call "多参数据转列表.vi"("参数名"="水中油", "测量数据块"=w293) -> ("添加的数组"=w291:string[][])  [unwired: 9 in]
                  n150 = Index Array(array=w291) -> (element #1=w290:string[], element #2=w289:string[])  [unwired: 4 in]
                  n151 = Insert Into Array(array=w296, new element=w289) -> (w295:string[][])  [unwired: 2 in]
                }
                frame 21 {
                  w306 = u16 21 items=["氨氮"=3, "水温"=9, "pH"=10, "溶解氧"=11, "电导率"=12, "浊度"=13, "叶绿素a"=14, "藻密度"=15, "蓝绿藻"=16, "氧化还原电位"=17, "溶解氧%"=18, "盐度"=19, "水中油"=20, "高锰酸盐指数"=21, "化学需氧量"=22, "比电导率"=23, "总溶解固体"=24, "pH电极电位"=25] ("下拉列表")
                  n152 = call "多参数测量数据读取.vi"("探头选择"=w306) -> ("测量数据块"=w302:T6)  [unwired: 8 in, 2 out]
                  n153 = call "多参数据转列表.vi"("参数名"="高锰酸盐指数", "测量数据块"=w302) -> ("添加的数组"=w301:string[][])  [unwired: 9 in]
                  n154 = Index Array(array=w301) -> (element #1=w299:string[], element #2=w298:string[])  [unwired: 4 in]
                  n155 = Insert Into Array(array=w305, new element=w298) -> (w304:string[][])  [unwired: 2 in]
                }
                frame 22 {
                  w315 = u16 22 items=["氨氮"=3, "水温"=9, "pH"=10, "溶解氧"=11, "电导率"=12, "浊度"=13, "叶绿素a"=14, "藻密度"=15, "蓝绿藻"=16, "氧化还原电位"=17, "溶解氧%"=18, "盐度"=19, "水中油"=20, "高锰酸盐指数"=21, "化学需氧量"=22, "比电导率"=23, "总溶解固体"=24, "pH电极电位"=25] ("下拉列表")
                  n156 = call "多参数测量数据读取.vi"("探头选择"=w315) -> ("测量数据块"=w311:T6)  [unwired: 8 in, 2 out]
                  n157 = call "多参数据转列表.vi"("参数名"="化学需氧量", "测量数据块"=w311) -> ("添加的数组"=w310:string[][])  [unwired: 9 in]
                  n158 = Index Array(array=w310) -> (element #1=w308:string[], element #2=w307:string[])  [unwired: 4 in]
                  n159 = Insert Into Array(array=w314, new element=w307) -> (w313:string[][])  [unwired: 2 in]
                }
              }
            }
            n160 = global write "多参数全局变量.vi" "传感器通道号"(w121) -> ()
            n161 = property on="数据区" class="MCListbox (严格)"("ColHdrString"=w127, "ItemNames"=w126) -> ()  [unwired: 2 in, 2 out]
          }
          frame Error {
          }
        }
      }
    }
  }
  n162 = property on="窗格" class="Pane"("Origin"=T2 {"Horizontal"=0, "Vertical"=0} ("原点")) -> ()  [unwired: 2 in, 2 out]
  n163 = property on="打开串口" class="Bool (严格)"("Val(Sgnl)"=TRUE ("值(信号)")) -> (error out=w1:errorcluster)  [unwired: 2 in, 1 out]
  n164 = Obtain Notifier(name (unnamed)="MPFlow" ("名称（未命名）"), notification data type=FALSE) -> (notifier out=w7:refnum<notifier>)  [unwired: 2 in, 2 out]
  n165 = control-ref of="控制命令区探头选择"() -> (w6:refnum<vi>)
  n166 = control-ref of="校准区探头选择"() -> (w3:refnum<vi>)
  n167 = control-ref of="K"() -> (w5:refnum<vi>)
  n168 = control-ref of="B"() -> (w4:refnum<vi>)
  n169 = while {
    tunnel: w8 -> [w321]
    tunnel: w7 -> [w320]
    tunnel: w6 -> [w319]
    tunnel: w5 -> [w318]
    tunnel: w4 -> [w317]
    tunnel: w3 -> [w316]
    tunnel: w1 -> [_]
    stop <- FALSE stop-if-true
    n170 = event shown="[9] \"测量数据区读取\": 值改变" {
      selector: _ -> [_ _ _ _ _ _ _ _ _ _ _ _ _ _ _ _ _ _ _ _]
      dyn-events: _ -> [_ _ _ _ _ _ _ _ _ _ _ _ _ _ _ _ _ _ _ _]
      timeout: _ -> [_ _ _ _ _ _ _ _ _ _ _ _ _ _ _ _ _ _ _ _]
      tunnel: w321 -> [_ _ _ w337 _ _ _ _ _ _ _ _ _ _ _ _ _ _ _ _]
      tunnel: w320 -> [_ _ _ _ w359 _ _ _ _ _ _ _ _ _ _ _ _ _ _ _]
      tunnel: w319 -> [_ _ _ _ _ _ _ _ _ _ _ _ _ _ _ w403 w410 _ _ _]
      tunnel: w318 -> [_ _ _ _ _ _ _ _ _ _ _ _ _ _ _ _ _ w416 _ _]
      tunnel: w317 -> [_ _ _ _ _ _ _ _ _ _ _ _ _ _ _ _ _ w418 _ _]
      tunnel: w316 -> [_ _ _ _ _ _ _ _ _ _ _ _ _ _ _ _ _ w420 _ w432]
      event Timeout {
        n171 = event-data() -> ()  [unwired: 1 in, 3 out]
      }
      event "释放串口": Value Change {
        n172 = event-data() -> ("NewVal"=w323:bool)  [unwired: 1 in, 5 out]
        n173 = case shown="真" w323 {
          frame False {
          }
          frame True {
            n174 = call "多参数通讯.vi"("STEP"=enum16{"open", "read", "write", "close"}."close") -> ("error out"=w324:errorcluster)  [unwired: 8 in, 2 out]
            n175 = case shown="无错误" w324 {
              frame No Error {
                n176 = property on="打开串口" class="Bool (严格)"("DisabledEnum"=T7."Enabled" ("禁用")) -> ()  [unwired: 2 in, 2 out]
              }
              frame Error {
              }
            }
          }
        }
      }
      event "打开串口": Value Change {
        n177 = event-data() -> ("NewVal"=w327:bool)  [unwired: 1 in, 5 out]
        n178 = case shown="真" w327 {
          frame False {
          }
          frame True {
            n179 = call "多参数通讯.vi"("STEP"=enum16{"open", "read", "write", "close"}."open") -> ("error out"=w328:errorcluster)  [unwired: 8 in, 2 out]
            n180 = case shown="错误" w328 {
              tunnel: [T7."Disabled and Grayed Out" ("禁用") T7."Enabled" ("禁用")] -> w330
              frame No Error {
              }
              frame Error {
                n181 = One Button Dialog(message="多参数串口打开失败" ("消息")) -> ()  [unwired: 1 in, 1 out]
              }
            }
            n182 = property on="打开串口" class="Bool (严格)"("DisabledEnum"=w330, "Value"=FALSE ("打开串口")) -> ()  [unwired: 2 in, 2 out]
          }
        }
      }
      event "手动启动": Value Change {
        n183 = event-data() -> ()  [unwired: 1 in, 6 out]
        n184 = call "多参数启动参数对话框.vi"() -> ("确认"=w336:bool, "测量时间"=w335:dbl)  [unwired: 10 in]
        n185 = case shown="真" w336 {
          tunnel: w337 -> [_ w339]
          tunnel: w335 -> [_ w338]
          frame False {
          }
          frame True {
            n186 = property class="VI"(reference=w339) -> ("Name"=w343:string, "Exec.State"=w341:T9)  [unwired: 1 in, 2 out]
            n187 = Open VI Reference(type specifier VI Refnum (for type only)=refnum<vi> refnum ("类型说明符VI引用句柄（仅用于类型）"), vi path=w343, options=128 ("选项")) -> (vi reference=w342:refnum<vi>)  [unwired: 3 in, 1 out]
            n188 = case shown="\"Idle\"" w341 {
              tunnel: w342 -> [w347 w354]
              tunnel: [w347 w353] -> w340
              tunnel: w338 -> [_ w348]
              frame "Bad", Default {
                n189 = One Button Dialog(message="仪器已经启动，无需重复启动" ("消息")) -> ()  [unwired: 1 in, 1 out]
              }
              frame "Idle" {
                n190 = global read "系统变量.vi" "运行模式"() -> (w350:enum16{"维护模式", "常规模式", "应急模式", "质控模式"})
                n191 = case shown="\"常规模式\", 默认" w350 {
                  tunnel: ["M" ("数据标记表") "hd" ("数据标记表")] -> w349
                  frame "维护模式" {
                  }
                  frame "常规模式", Default {
                  }
                }
                n192 = Bundle By Name(cluster=T8 {"测量模式"=enum."水样测试", "数据标记表"="", "测量时间"=0.0} ("启动参数"), "数据标记表"=w349, "测量时间"=w348) -> (w351:T8)
                n193 = call-by-ref "开始异步调用"(reference=w354, "启动参数"=w351) -> (reference out=w353:refnum<vi>)  [unwired: 12 in, 1 out]
              }
            }
            n194 = Close Reference(reference=w340) -> ()  [unwired: 1 in, 1 out]
          }
        }
      }
      event "停止": Value Change {
        n195 = event-data() -> ()  [unwired: 1 in, 6 out]
        n196 = Two Button Dialog(message="请再一次确认是否停止测量" ("消息")) -> (T button?=w357:bool)  [unwired: 2 in]
        n197 = case shown="真" w357 {
          tunnel: w359 -> [_ w362]
          frame False {
          }
          frame True {
            w360 = u16 11 items=["启动测量（全部）"=1, "初始化（清洗）"=10, "停止测量（全部）"=11, "校时"=13, "启动测量（单个传感器）"=19, "停止测量（单个传感器）"=20] ("控制命令")
            w361 = u16 10 items=["氨氮"=3, "水温"=9, "pH值"=10, "溶解氧"=11, "电导率"=12, "浊度"=13, "叶绿素a"=14, "藻密度"=15, "蓝绿藻"=16, "氧化还原电位"=17, "溶解氧%"=18, "盐度"=19] ("站号")
            n198 = Send Notification(notification=TRUE ("通知"), notifier=w362) -> ()  [unwired: 1 in, 2 out]
            n199 = call "多参数控制命令.vi"("控制命令"=w360, "站号"=w361) -> ()  [unwired: 9 in, 1 out]
          }
        }
      }
      event "设置": Value Change {
        n200 = event-data() -> ()  [unwired: 1 in, 6 out]
        n201 = property on="窗格" class="Pane"("Origin"=T2 {"Horizontal"=0, "Vertical"=628} ("原点")) -> ()  [unwired: 2 in, 2 out]
      }
      event "返回": Value Change {
        n202 = event-data() -> ()  [unwired: 1 in, 6 out]
        n203 = property on="窗格" class="Pane"("Origin"=T2 {"Horizontal"=0, "Vertical"=0} ("原点")) -> ()  [unwired: 2 in, 2 out]
      }
      event "传感器参数读取": Value Change {
        n204 = event-data() -> ()  [unwired: 1 in, 6 out]
        n205 = call "多参数传感器参数读取.vi"() -> ("error out"=w366:errorcluster, "添加的数组"=w367:string[][])  [unwired: 10 in]
        n206 = call <vilib>:"General Error Handler.vi"("error in (no error)"=w366) -> ()  [unwired: 10 in, 5 out]
        n207 = property on="传感器区" class="MCListbox (严格)"("ItemNames"=w367) -> ()  [unwired: 2 in, 2 out]
      }
      event "关键参数区读取": Value Change {
        n208 = event-data() -> ()  [unwired: 1 in, 6 out]
        n209 = call "多参数关键参数读取.vi"() -> ("error out"=w368:errorcluster, "添加的数组"=w369:string[][])  [unwired: 10 in]
        n210 = call <vilib>:"General Error Handler.vi"("error in (no error)"=w368) -> ()  [unwired: 10 in, 5 out]
        n211 = property on="关键参数区" class="MCListbox (严格)"("ItemNames"=w369) -> ()  [unwired: 2 in, 2 out]
      }
      event "测量数据区读取": Value Change {
        n212 = event-data() -> ()  [unwired: 1 in, 6 out]
        n213 = call "多参数测量数据读取.vi"("探头选择"="探头选择") -> ("error out"=w372:errorcluster, "添加的数组"=w370:string[][])  [unwired: 8 in, 1 out]
        n214 = call <vilib>:"General Error Handler.vi"("error in (no error)"=w372) -> ()  [unwired: 10 in, 5 out]
        n215 = property on="测量数据区" class="MCListbox (严格)"("ItemNames"=w370) -> ()  [unwired: 2 in, 2 out]
      }
      event "状态告警区读取": Value Change {
        n216 = event-data() -> ()  [unwired: 1 in, 6 out]
        n217 = call "多参数状态告警区读取.vi"() -> ("error out"=w373:errorcluster, "添加的数组"=w374:string[][])  [unwired: 9 in, 1 out]
        n218 = call <vilib>:"General Error Handler.vi"("error in (no error)"=w373) -> ()  [unwired: 10 in, 5 out]
        n219 = property on="状态告警区" class="MCListbox (严格)"("ItemNames"=w374) -> ()  [unwired: 2 in, 2 out]
      }
      event "同步时间": Value Change {
        w375 = u16 13 items=["启动测量（全部）"=1, "初始化（清洗）"=10, "停止测量（全部）"=11, "校时"=13, "启动测量（单个传感器）"=19, "停止测量（单个传感器）"=20] ("控制命令")
        w376 = u16 9 items=["氨氮"=3, "水温"=9, "pH值"=10, "溶解氧"=11, "电导率"=12, "浊度"=13, "叶绿素a"=14, "藻密度"=15, "蓝绿藻"=16, "氧化还原电位"=17, "溶解氧%"=18, "盐度"=19] ("站号")
        n220 = event-data() -> ()  [unwired: 1 in, 6 out]
        n221 = call "多参数控制命令.vi"("控制命令"=w375, "站号"=w376) -> ("error out"=w378:errorcluster)  [unwired: 9 in]
        n222 = case shown="错误" w378 {
          tunnel: ["时间同步成功" ("消息") "时间同步失败" ("消息")] -> w377
          frame No Error {
          }
          frame Error {
          }
        }
        n223 = One Button Dialog(message=w377) -> ()  [unwired: 1 in, 1 out]
      }
      event "启动测量(全部)": Value Change {
        w381 = u16 1 items=["启动测量（全部）"=1, "初始化（清洗）"=10, "停止测量（全部）"=11, "校时"=13, "启动测量（单个传感器）"=19, "停止测量（单个传感器）"=20] ("控制命令")
        w382 = u16 9 items=["氨氮"=3, "水温"=9, "pH值"=10, "溶解氧"=11, "电导率"=12, "浊度"=13, "叶绿素a"=14, "藻密度"=15, "蓝绿藻"=16, "氧化还原电位"=17, "溶解氧%"=18, "盐度"=19] ("站号")
        n224 = event-data() -> ()  [unwired: 1 in, 6 out]
        n225 = call "多参数控制命令.vi"("控制命令"=w381, "站号"=w382) -> ("error out"=w384:errorcluster)  [unwired: 9 in]
        n226 = case shown="无错误" w384 {
          tunnel: ["启动成功" ("消息") "启动失败" ("消息")] -> w383
          frame No Error {
          }
          frame Error {
          }
        }
        n227 = One Button Dialog(message=w383) -> ()  [unwired: 1 in, 1 out]
      }
      event "停止测量(全部)": Value Change {
        w389 = u16 11 items=["启动测量（全部）"=1, "初始化（清洗）"=10, "停止测量（全部）"=11, "校时"=13, "启动测量（单个传感器）"=19, "停止测量（单个传感器）"=20] ("控制命令")
        w390 = u16 9 items=["氨氮"=3, "水温"=9, "pH值"=10, "溶解氧"=11, "电导率"=12, "浊度"=13, "叶绿素a"=14, "藻密度"=15, "蓝绿藻"=16, "氧化还原电位"=17, "溶解氧%"=18, "盐度"=19] ("站号")
        n228 = event-data() -> ()  [unwired: 1 in, 6 out]
        n229 = call "多参数控制命令.vi"("控制命令"=w389, "站号"=w390) -> ("error out"=w388:errorcluster)  [unwired: 9 in]
        n230 = case shown="错误" w388 {
          tunnel: ["停止成功" ("消息") "停止失败" ("消息")] -> w387
          frame No Error {
          }
          frame Error {
          }
        }
        n231 = One Button Dialog(message=w387) -> ()  [unwired: 1 in, 1 out]
      }
      event "初始化(清洗)": Value Change {
        w395 = u16 10 items=["启动测量（全部）"=1, "初始化（清洗）"=10, "停止测量（全部）"=11, "校时"=13, "启动测量（单个传感器）"=19, "停止测量（单个传感器）"=20] ("控制命令")
        w396 = u16 9 items=["氨氮"=3, "水温"=9, "pH值"=10, "溶解氧"=11, "电导率"=12, "浊度"=13, "叶绿素a"=14, "藻密度"=15, "蓝绿藻"=16, "氧化还原电位"=17, "溶解氧%"=18, "盐度"=19] ("站号")
        n232 = event-data() -> ()  [unwired: 1 in, 6 out]
        n233 = call "多参数控制命令.vi"("控制命令"=w395, "站号"=w396) -> ("error out"=w393:errorcluster)  [unwired: 9 in]
        n234 = case shown="错误" w393 {
          tunnel: ["初始化成功" ("消息") "初始化失败" ("消息")] -> w394
          frame No Error {
          }
          frame Error {
          }
        }
        n235 = One Button Dialog(message=w394) -> ()  [unwired: 1 in, 1 out]
      }
      event "启动测量(单探)": Value Change {
        w399 = u16 19 items=["启动测量（全部）"=1, "初始化（清洗）"=10, "停止测量（全部）"=11, "校时"=13, "启动测量（单个传感器）"=19, "停止测量（单个传感器）"=20] ("控制命令")
        n236 = event-data() -> ()  [unwired: 1 in, 6 out]
        n237 = property class="Ring (严格)"(reference=w403) -> ("Value"=w402:u16)  [unwired: 1 in, 2 out]
        n238 = call "多参数控制命令.vi"("控制命令"=w399, "站号"=w402) -> ("error out"=w401:errorcluster)  [unwired: 9 in]
        n239 = case shown="无错误" w401 {
          tunnel: ["启动成功" ("消息") "启动失败" ("消息")] -> w400
          frame No Error {
          }
          frame Error {
          }
        }
        n240 = One Button Dialog(message=w400) -> ()  [unwired: 1 in, 1 out]
      }
      event "停止测量(单探)": Value Change {
        w406 = u16 20 items=["启动测量（全部）"=1, "初始化（清洗）"=10, "停止测量（全部）"=11, "校时"=13, "启动测量（单个传感器）"=19, "停止测量（单个传感器）"=20] ("控制命令")
        n241 = event-data() -> ()  [unwired: 1 in, 6 out]
        n242 = property class="Ring (严格)"(reference=w410) -> ("Value"=w409:u16)  [unwired: 1 in, 2 out]
        n243 = call "多参数控制命令.vi"("控制命令"=w406, "站号"=w409) -> ("error out"=w408:errorcluster)  [unwired: 9 in]
        n244 = case shown="错误" w408 {
          tunnel: ["停止成功" ("消息") "停止失败" ("消息")] -> w407
          frame No Error {
          }
          frame Error {
          }
        }
        n245 = One Button Dialog(message=w407) -> ()  [unwired: 1 in, 1 out]
      }
      event "写入KB": Value Change {
        n246 = event-data() -> ()  [unwired: 1 in, 6 out]
        n247 = property class="DigNum (严格)"(reference=w416) -> ("Value"=w415:dbl)  [unwired: 1 in, 2 out]
        n248 = property class="DigNum (严格)"(reference=w418) -> ("Value"=w417:dbl)  [unwired: 1 in, 2 out]
        n249 = property class="Ring (严格)"(reference=w420) -> ("Value"=w419:u16)  [unwired: 1 in, 2 out]
        n250 = call "多参数校准写入.vi"("B"=w417, "K"=w415, "站号"=w419) -> ("error out"=w413:errorcluster)  [unwired: 8 in]
        n251 = case shown="错误" w413 {
          tunnel: ["写入成功" ("消息") "写入失败" ("消息")] -> w414
          frame No Error {
          }
          frame Error {
          }
        }
        n252 = One Button Dialog(message=w414) -> ()  [unwired: 1 in, 1 out]
      }
      event "K", "B": Mouse Down {
        n253 = event-data() -> ("CtlRef"=w426:refnum<vi>)  [unwired: 1 in, 5 out]
        n254 = property class="DigNum (严格)"(reference=w426) -> (reference out=w425:refnum<vi>, "Value"=w424:dbl)  [unwired: 1 in, 1 out]
        n255 = call "数字键盘.vi"("OldNumber"=w424) -> ("NewNumber"=w423:sgl)
        n256 = property class="DigNum (严格)"(reference=w425, "Value"=w423) -> ()  [unwired: 1 in, 2 out]
      }
      event "读取KB": Value Change {
        n257 = event-data() -> ()  [unwired: 1 in, 6 out]
        n258 = property class="Ring (严格)"(reference=w432) -> ("Value"=w431:u16)  [unwired: 1 in, 2 out]
        n259 = call "多参校准读取.vi"("站号"=w431) -> ("error out"=w427:errorcluster, "B"=→"B":dbl, "K"=→"K":dbl)  [unwired: 8 in]
        n260 = case shown="无错误" w427 {
          tunnel: ["读取成功" ("消息") "读取失败" ("消息")] -> w428
          frame No Error {
          }
          frame Error {
          }
        }
        n261 = One Button Dialog(message=w428) -> ()  [unwired: 1 in, 1 out]
      }
    }
  }
